vi "Update Popup Image Window Name.vi"(8 "error in (no error)":errorcluster, 10 "Window Name":string, 11 "UI in":refnum<class "UI.lvclass">) -> (0 "error out":errorcluster)   [LabVIEW 2020, in "AR Example.lvlib" / "UI.lvclass"]
uses:
  UI.lvclass
  UI.lvclass/UI.ctl
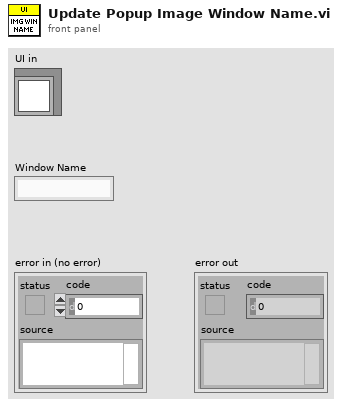
[diagram p1: front panel]
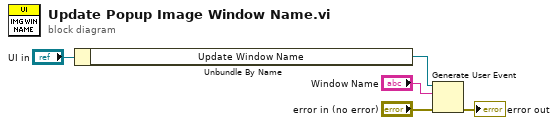
[diagram p0: block diagram]
diagram:
  n1 = Unbundle By Name("UI in") -> ("Update Window Name"=w4:refnum<user-event>)
  n2 = Generate User Event(user event=w4, event data cluster="Window Name", error in="error in (no error)") -> (error out=→"error out":errorcluster)  [unwired: 1 in, 1 out]
